vi "Wrapper.vi"   [LabVIEW 2009]
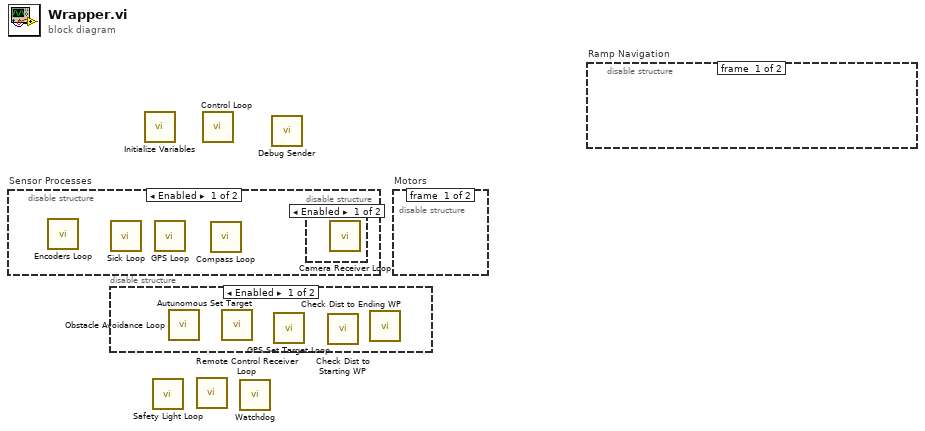
[diagram p0: block diagram]
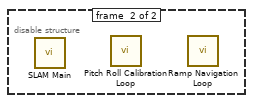
[diagram p2: hidden frame]
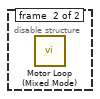
[diagram p6: hidden frame]
diagram:
  n1 = disable-structure "Sensor Processes" shown="Enabled" {
    frame #0 {
      n2 = call "Encoders Loop.vi"() -> ()  [unwired: 1 in]
      n3 = call "Sick Loop.vi"() -> ()  [unwired: 1 in]
      n4 = call "GPS Loop.vi"() -> ()  [unwired: 1 in]
      n5 = call "Compass Loop.vi"() -> ()  [unwired: 1 in]
      n6 = disable-structure shown="Enabled" {
        frame #0 {
          n7 = call "Camera Receiver Loop.vi"() -> ()  [unwired: 1 in]
        }
        frame #1 {
        }
      }
    }
    frame #1 {
    }
  }
  n8 = disable-structure shown="Enabled" {
    frame #0 {
      n9 = call "Obstacle Avoidance Loop.vi"() -> ()  [unwired: 1 in]
      n10 = call "Autunomous Set Target.vi"() -> ()  [unwired: 12 in]
      n11 = call "GPS Set Target Loop.vi"() -> ()  [unwired: 1 in]
      n12 = call "Check Dist to Starting WP.vi"() -> ()  [unwired: 1 in]
      n13 = call "Check Dist to Ending WP.vi"() -> ()  [unwired: 1 in]
    }
    frame #1 {
    }
  }
  n14 = call "Initialize Variables.vi"() -> ()  [unwired: 1 in]
  n15 = call "Safety Light Loop.vi"() -> ()  [unwired: 1 in]
  n16 = call "Remote Control Receiver Loop.vi"() -> ()  [unwired: 1 in]
  n17 = call "Control Loop.vi"() -> ()  [unwired: 1 in]
  n18 = call "Watchdog.vi"() -> ()  [unwired: 1 in]
  n19 = call "Debug Sender.vi"() -> ()  [unwired: 1 in]
  n20 = disable-structure "Motors" shown="Enabled" {
    frame #0 {
    }
    frame #1 {
      n21 = call "Motor Loop (Mixed Mode).vi"() -> ()  [unwired: 1 in]
    }
  }
  n22 = disable-structure "Ramp Navigation" shown="Disabled" {
    frame #0 {
    }
    frame #1 {
      n23 = call "SLAM Main.vi"() -> ()  [unwired: 12 in]
      n24 = call "Pitch Roll Calibration Loop.vi"() -> ()  [unwired: 1 in]
      n25 = call "Ramp Navigation Loop.vi"() -> ()  [unwired: 1 in]
    }
  }
